vi "Configure Display Offset.vi"(7 "Measurement Number (1: Measurement 1)":i32(ring)=1 items=["Measurement 1"=1, "Measurement 2"=2, "Measurement 3"=3, "Measurement 4"=4], 8 "error in (no error)":errorcluster, 9 "Display Offset (0 dB)":dbl, 10 "Enable Display Offset (F: Disable)":bool, 11 "VISA resource name":refnum<visa-resource-name>) -> (0 "error out":errorcluster, 3 "VISA resource name out":refnum<visa-resource-name>)   [LabVIEW 2011, in "Agilent N432A.lvlib"]
doc: "Configures the display offset value on the specified window/measurement. A display offset is applied to the measured power after any channel offset or mathematical functions have been included."
uses:
  <instrlib>/Agilent N432A/Agilent N432A.lvlib
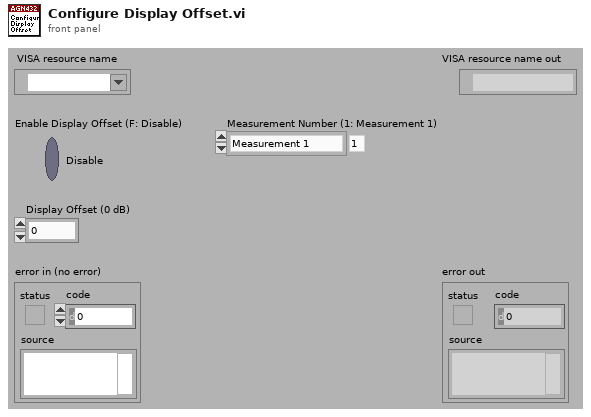
[diagram p1: front panel]
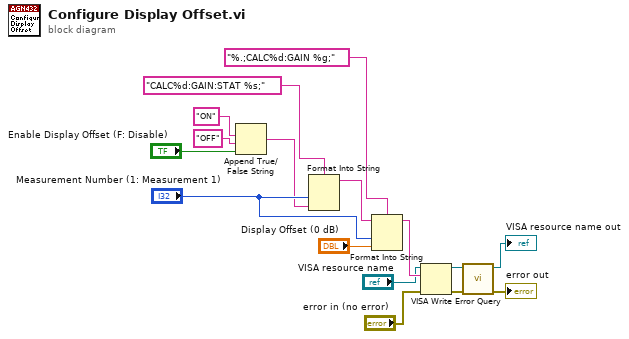
[diagram p0: block diagram]
diagram:
  n1 = Append True/False String(1:"Enable Display Offset (F: Disable)", 2:"OFF", 3:"ON") -> (0:w11:string)  [unwired: 1 in]
  n2 = Format Into String(format string="CALC%d:GAIN:STAT %s;", "Measurement Number (1: Measurement 1)", w11) -> (resulting string=w10:string)  [unwired: 2 in, 1 out]
  n3 = Format Into String(format string="%.;CALC%d:GAIN %g;", initial string=w10, "Measurement Number (1: Measurement 1)", "Display Offset (0 dB)") -> (resulting string=w7:string)  [unwired: 1 in, 1 out]
  n4 = VISA Write(VISA resource name="VISA resource name", write buffer=w7, error in (no error)="error in (no error)") -> (VISA resource name out=w4:refnum<visa-resource-name>, error out=w3:errorcluster)  [unwired: 1 out]
  n5 = call <instrlib>:"Error Query.vi"("error in (no error)"=w3, "VISA resource name"=w4) -> ("error out"=→"error out":errorcluster, "VISA resource name out"=→"VISA resource name out":refnum<visa-resource-name>)  [unwired: 6 in, 2 out]
